vi "Set Control.vi"(8 "error in (no error)":errorcluster, 9 "Output #":i32=1, 10 "Control":T1, 11 "Cryo-Con Driver in":refnum<class "Cryo-Con Driver.lvclass">) -> (0 "error out":errorcluster, 3 "Cryo-Con Driver out":refnum<class "Cryo-Con Driver.lvclass">)   [LabVIEW 2021, in "Cryo-Con Driver.lvclass"]
uses:
  Cryo-Con Driver.lvclass
  C:/GitHub/NHMFL_Core/Libraries/Instruments/VISA Instrument/VISA Instrument.lvclass
  C:/GitHub/NHMFL_Core/Libraries/Instruments/Temperature Controller Driver/Temperature Controller Driver.lvclass
  Temperature Controller/Controls/Control Mode.ctl
  VISA Instrument/VISA Instrument.lvclass/VISA Instrument.ctl
  VISA Instrument/Read VISA resource.vi
  VISA Instrument/Write VISA resource.vi
  Temperature Controller Driver/Read T controller configuration.vi
  Cryo-Con Driver.lvclass/Cryo-Con Driver.ctl
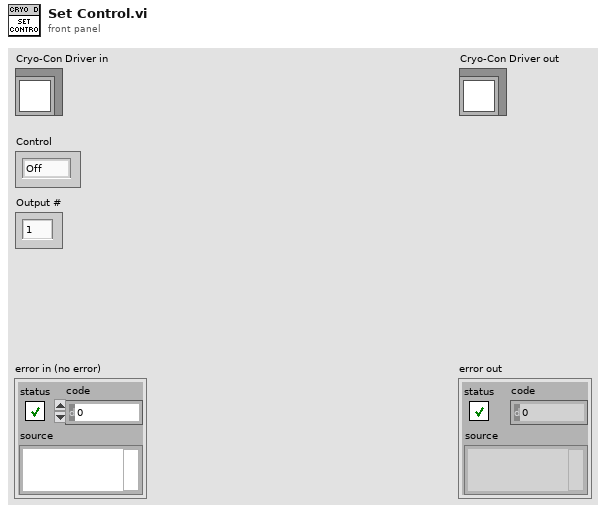
[diagram p1: front panel]
types:
  T1 = typedef "Control Mode.ctl" = enum16{"Off", "PID", "Ramp", "Manual", "Table"}
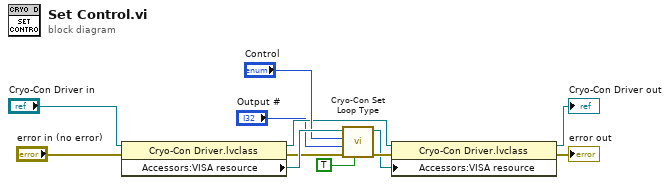
[diagram p0: block diagram]
diagram:
  n1 = property class="Cryo-Con Driver.lvclass"(reference="Cryo-Con Driver in", error in="error in (no error)") -> (reference out=w7:refnum<class "Cryo-Con Driver.lvclass">, error out=w9:errorcluster, "Accessors:VISA resource"=w10:refnum<visa-resource-name>)
  n2 = call "Cryo-Con Set Loop Type.vi"("Change control state"=TRUE, "error in (no error)"=w9, "Loop number"="Output #", "Set T"="Control", "VISA Resource Name"=w10) -> ("error out"=w4:errorcluster, "VISA Resource Name Out"=w3:refnum<visa-resource-name>)  [unwired: 5 in]
  n3 = property class="Cryo-Con Driver.lvclass"(reference=w7, error in=w4, "Accessors:VISA resource"=w3) -> (reference out=→"Cryo-Con Driver out":refnum<class "Cryo-Con Driver.lvclass">, error out=→"error out":errorcluster)
